vi "read data.vi"(0 "Control ref":refnum<vi>, 2 "Data In":T1, 4 "index":i32, 5 "error in (no error)":errorcluster) -> ()   [LabVIEW 2014, in "X DIM conditions.xctl"]
uses:
  X DIM conditions.xctl
  X DIM conditions.Data.ctl
  PTSequencer/PTSequencer.DIM service condition.ctl
  CSCore/CSSystem/CoreDefs/CoreDefs.rawDataType.ctl
  CSCore/CSSystem/CoreLib/CoreLib.byte array 2 string.vi
  CSCore/CSSystem/CoreLib/CoreLib.byte array 2 int.vi
  CSCore/CSSystem/CoreLib/CoreLib.byte array 2 int array.vi
  CSCore/CSSystem/CoreLib/CoreLib.byte array 2 short.vi
  CSCore/CSSystem/CoreLib/CoreLib.byte array 2 short array.vi
  CSCore/CSSystem/CoreLib/CoreLib.byte array 2 double.vi
  CSCore/CSSystem/CoreLib/CoreLib.byte array 2 double array.vi
  CSCore/CSSystem/CoreLib/CoreLib.byte array 2 float.vi
  CSCore/CSSystem/CoreLib/CoreLib.byte array 2 float array.vi
  CSCore/CSSystem/CoreLib/CoreLib.lvlib
  PTSequencer/PTSequencer.lvlib
panel:
  in  "Control":T4
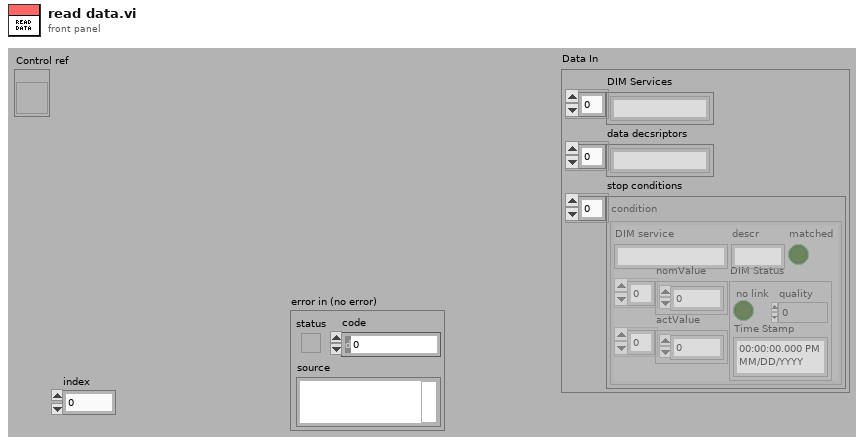
[diagram p1: front panel]
types:
  T1 = typedef "X DIM conditions.xctl/X DIM conditions.Data.ctl" = cluster{"DIM Services":string[], "data decsriptors":string[], "stop conditions":T2[]}
  T2 = typedef "PTSequencer.lvlib/PTSequencer.DIM service condition.ctl" = cluster{"DIM service":string, "descr":string, "nomValue":T3, "actValue":T3, "matched":bool, "DIM Status":cluster{"no link":bool, "quality":i32, "Time Stamp":timestamp}}
  T3 = typedef "CoreDefs.rawDataType.ctl" = i8[]
  T4 = cluster{"Name 1":u16, "Descr 1":string, "Value 1":string, "Used 1":bool, "Name 2":u16, "Descr 2":string, "Value 2":string, "Used 2":bool, "Name 3":u16, "Descr 3":string, "Value 3":string, "Used 3":bool, "Name 4":u16, "Descr 4":string, "Value 4":string, "Used 4":bool}
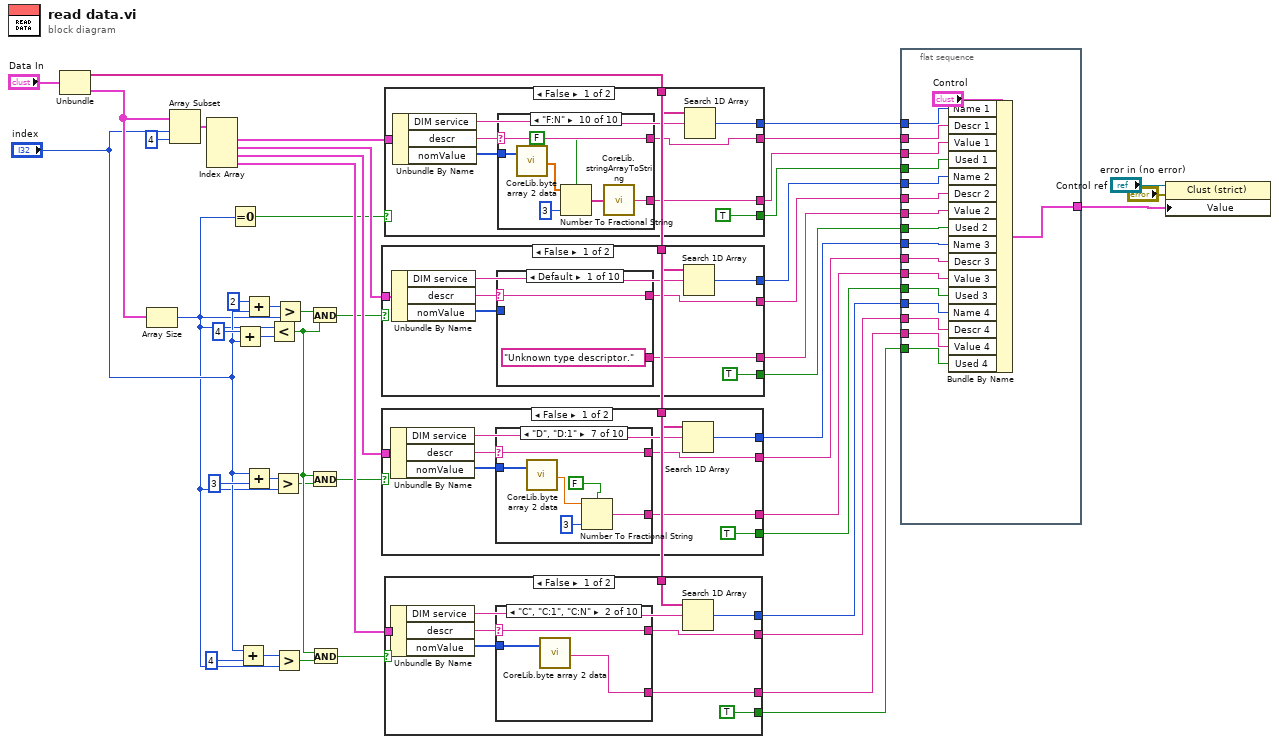
[diagram p0: block diagram]
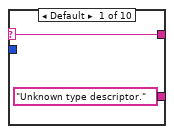
[diagram p2: hidden frame]
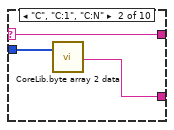
[diagram p3: hidden frame]
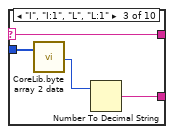
[diagram p4: hidden frame]
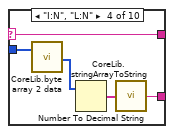
[diagram p5: hidden frame]
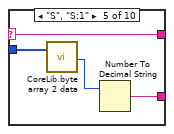
[diagram p6: hidden frame]
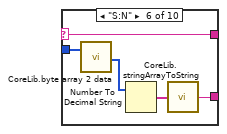
[diagram p7: hidden frame]
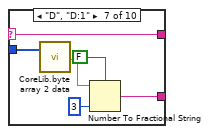
[diagram p8: hidden frame]
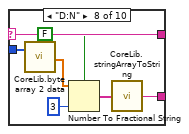
[diagram p9: hidden frame]
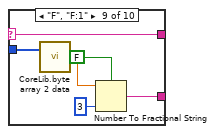
[diagram p10: hidden frame]
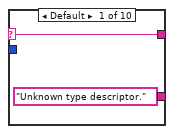
[diagram p12: hidden frame]
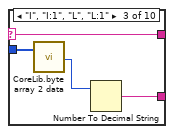
[diagram p13: hidden frame]
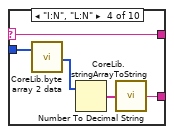
[diagram p14: hidden frame]
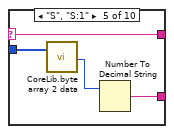
[diagram p15: hidden frame]
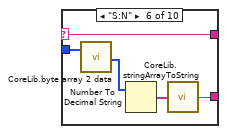
[diagram p16: hidden frame]
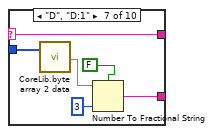
[diagram p17: hidden frame]
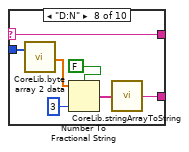
[diagram p18: hidden frame]
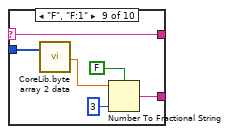
[diagram p19: hidden frame]
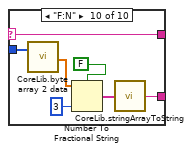
[diagram p20: hidden frame]
diagram:
  n1 = Unbundle("Data In") -> ("DIM Services"=w24:string[], "stop conditions"=w23:T2[])  [unwired: 1 out]
  n2 = Array Size(array=w23) -> (size(s)=w2:i32)
  n3 = Array Subset(array=w23, index="index", length=4) -> (w45:T2[])
  n4 = Index Array(array=w45) -> (element #1=w44:T2, element #2=w43:T2, element #3=w42:T2, element #4=w41:T2)  [unwired: 4 in]
  n5 = Equal To 0?(x=w2) -> (x = 0?=w1:bool)
  n6 = Add(x=4, y="index") -> (x+y=w15:i32)
  n7 = Add(x="index", y=4) -> (x+y=w19:i32)
  n8 = Add(x=2, y="index") -> (x+y=w16:i32)
  n9 = Add(x="index", y=3) -> (x+y=w18:i32)
  n10 = Less?(x=w2, y=w15) -> (x < y?=w13:bool)
  n11 = Greater?(x=w18, y=w2) -> (0:w11:bool)
  n12 = Greater?(x=w19, y=w2) -> (0:w12:bool)
  n13 = Greater?(x=w16, y=w2) -> (0:w10:bool)
  n14 = And(x=w10, y=w13) -> (x .and. y?=w6:bool)
  n15 = And(x=w13, y=w11) -> (x .and. y?=w7:bool)
  n16 = And(x=w13, y=w12) -> (x .and. y?=w8:bool)
  n17 = case shown="False" w6 {
    tunnel: w43 -> [w52 _]
    tunnel: [w51 _] -> w39
    tunnel: [w50 _] -> w37
    tunnel: [w49 _] -> w36
    tunnel: w24 -> [w48 _]
    tunnel: [TRUE _] -> w5
    frame False {
      n18 = Unbundle By Name(w52) -> ("DIM service"=w55:string, "descr"=w53:string, "nomValue"=w54:T3)
      n19 = case shown="Default" w53 {
        selector: w53 -> [w56 w58 w61 w65 w70 w74 w83 w87 w96 w100]
        tunnel: w54 -> [_ w60 w64 w69 w73 w78 w84 w91 w97 w102]
        tunnel: ["Unknown type descriptor." w59 w62 w66 w71 w75 w81 w88 w94 w101] -> w49
        tunnel: [w56 w58 w61 w65 w70 w74 w83 w87 w96 w100] -> w50
        frame Default {
        }
        frame "C", "C:1", "C:N" {
          n20 = call-poly "CoreLib.byte array 2 data.vi"("byteArray"=w60) -> ("string"=w59:string)  [unwired: 16 in, 2 out]
        }
        frame "I", "I:1", "L", "L:1" {
          n21 = call-poly "CoreLib.byte array 2 data.vi"("byteArray"=w64) -> ("i32"=w63:i32)  [unwired: 16 in, 2 out]
          n22 = Number To Decimal String(number=w63) -> (decimal integer string=w62:string)  [unwired: 1 in]
        }
        frame "I:N", "L:N" {
          n23 = call-poly "CoreLib.byte array 2 data.vi"("byteArray"=w69) -> ("[i32]"=w68:i32[])  [unwired: 16 in, 2 out]
          n24 = Number To Decimal String(number=w68) -> (decimal integer string=w67:string[])  [unwired: 1 in]
          n25 = call "CoreLib.stringArrayToString.vi"("Array"=w67) -> ("String"=w66:string)
        }
        frame "S", "S:1" {
          n26 = call-poly "CoreLib.byte array 2 data.vi"("byteArray"=w73) -> ("i16"=w72:i16)  [unwired: 16 in, 2 out]
          n27 = Number To Decimal String(number=w72) -> (decimal integer string=w71:string)  [unwired: 1 in]
        }
        frame "S:N" {
          n28 = call-poly "CoreLib.byte array 2 data.vi"("byteArray"=w78) -> ("[i16]"=w77:i16[])  [unwired: 16 in, 2 out]
          n29 = Number To Decimal String(number=w77) -> (decimal integer string=w76:string[])  [unwired: 1 in]
          n30 = call "CoreLib.stringArrayToString.vi"("Array"=w76) -> ("String"=w75:string)
        }
        frame "D", "D:1" {
          n31 = call-poly "CoreLib.byte array 2 data.vi"("byteArray"=w84) -> ("d64"=w80:dbl)  [unwired: 16 in, 2 out]
          n32 = Number To Fractional String(use system decimal point (T)=FALSE, number=w80, precision (6)=i16 3) -> (F-format string=w81:string)  [unwired: 1 in]
        }
        frame "D:N" {
          n33 = call-poly "CoreLib.byte array 2 data.vi"("byteArray"=w91) -> ("[d64]"=w90:dbl[])  [unwired: 16 in, 2 out]
          n34 = Number To Fractional String(use system decimal point (T)=FALSE, number=w90, precision (6)=i16 3) -> (F-format string=w89:string[])  [unwired: 1 in]
          n35 = call "CoreLib.stringArrayToString.vi"("Array"=w89) -> ("String"=w88:string)
        }
        frame "F", "F:1" {
          n36 = call-poly "CoreLib.byte array 2 data.vi"("byteArray"=w97) -> ("f32"=w93:sgl)  [unwired: 16 in, 2 out]
          n37 = Number To Fractional String(use system decimal point (T)=FALSE, number=w93, precision (6)=i16 3) -> (F-format string=w94:string)  [unwired: 1 in]
        }
        frame "F:N" {
          n38 = call-poly "CoreLib.byte array 2 data.vi"("byteArray"=w102) -> ("[f32]"=w104:sgl[])  [unwired: 16 in, 2 out]
          n39 = Number To Fractional String(use system decimal point (T)=FALSE, number=w104, precision (6)=i16 3) -> (F-format string=w103:string[])  [unwired: 1 in]
          n40 = call "CoreLib.stringArrayToString.vi"("Array"=w103) -> ("String"=w101:string)
        }
      }
      n41 = Search 1D Array(1D array=w48, element=w55) -> (index of element=w51:i32)  [unwired: 1 in]
    }
    frame True {
    }
  }
  n42 = case shown="False" w7 {
    tunnel: w42 -> [w110 _]
    tunnel: [w109 _] -> w38
    tunnel: [w108 _] -> w35
    tunnel: [w107 _] -> w34
    tunnel: w24 -> [w106 _]
    tunnel: [TRUE _] -> w4
    frame False {
      n43 = Unbundle By Name(w110) -> ("DIM service"=w111:string, "descr"=w113:string, "nomValue"=w112:T3)
      n44 = case shown="\"D\", \"D:1\"" w113 {
        selector: w113 -> [w114 w116 w119 w123 w128 w132 w141 w145 w154 w158]
        tunnel: w112 -> [_ w118 w122 w127 w131 w136 w142 w149 w155 w160]
        tunnel: ["Unknown type descriptor." w117 w120 w124 w129 w133 w138 w146 w152 w159] -> w107
        tunnel: [w114 w116 w119 w123 w128 w132 w141 w145 w154 w158] -> w108
        frame Default {
        }
        frame "C", "C:1", "C:N" {
          n45 = call-poly "CoreLib.byte array 2 data.vi"("byteArray"=w118) -> ("string"=w117:string)  [unwired: 16 in, 2 out]
        }
        frame "I", "I:1", "L", "L:1" {
          n46 = call-poly "CoreLib.byte array 2 data.vi"("byteArray"=w122) -> ("i32"=w121:i32)  [unwired: 16 in, 2 out]
          n47 = Number To Decimal String(number=w121) -> (decimal integer string=w120:string)  [unwired: 1 in]
        }
        frame "I:N", "L:N" {
          n48 = call-poly "CoreLib.byte array 2 data.vi"("byteArray"=w127) -> ("[i32]"=w126:i32[])  [unwired: 16 in, 2 out]
          n49 = Number To Decimal String(number=w126) -> (decimal integer string=w125:string[])  [unwired: 1 in]
          n50 = call "CoreLib.stringArrayToString.vi"("Array"=w125) -> ("String"=w124:string)
        }
        frame "S", "S:1" {
          n51 = call-poly "CoreLib.byte array 2 data.vi"("byteArray"=w131) -> ("i16"=w130:i16)  [unwired: 16 in, 2 out]
          n52 = Number To Decimal String(number=w130) -> (decimal integer string=w129:string)  [unwired: 1 in]
        }
        frame "S:N" {
          n53 = call-poly "CoreLib.byte array 2 data.vi"("byteArray"=w136) -> ("[i16]"=w135:i16[])  [unwired: 16 in, 2 out]
          n54 = Number To Decimal String(number=w135) -> (decimal integer string=w134:string[])  [unwired: 1 in]
          n55 = call "CoreLib.stringArrayToString.vi"("Array"=w134) -> ("String"=w133:string)
        }
        frame "D", "D:1" {
          n56 = call-poly "CoreLib.byte array 2 data.vi"("byteArray"=w142) -> ("d64"=w139:dbl)  [unwired: 16 in, 2 out]
          n57 = Number To Fractional String(use system decimal point (T)=FALSE, number=w139, precision (6)=i16 3) -> (F-format string=w138:string)  [unwired: 1 in]
        }
        frame "D:N" {
          n58 = call-poly "CoreLib.byte array 2 data.vi"("byteArray"=w149) -> ("[d64]"=w148:dbl[])  [unwired: 16 in, 2 out]
          n59 = Number To Fractional String(use system decimal point (T)=FALSE, number=w148, precision (6)=i16 3) -> (F-format string=w147:string[])  [unwired: 1 in]
          n60 = call "CoreLib.stringArrayToString.vi"("Array"=w147) -> ("String"=w146:string)
        }
        frame "F", "F:1" {
          n61 = call-poly "CoreLib.byte array 2 data.vi"("byteArray"=w155) -> ("f32"=w151:sgl)  [unwired: 16 in, 2 out]
          n62 = Number To Fractional String(use system decimal point (T)=FALSE, number=w151, precision (6)=i16 3) -> (F-format string=w152:string)  [unwired: 1 in]
        }
        frame "F:N" {
          n63 = call-poly "CoreLib.byte array 2 data.vi"("byteArray"=w160) -> ("[f32]"=w162:sgl[])  [unwired: 16 in, 2 out]
          n64 = Number To Fractional String(use system decimal point (T)=FALSE, number=w162, precision (6)=i16 3) -> (F-format string=w161:string[])  [unwired: 1 in]
          n65 = call "CoreLib.stringArrayToString.vi"("Array"=w161) -> ("String"=w159:string)
        }
      }
      n66 = Search 1D Array(1D array=w106, element=w111) -> (index of element=w109:i32)  [unwired: 1 in]
    }
    frame True {
    }
  }
  n67 = case shown="False" w1 {
    tunnel: w44 -> [w168 _]
    tunnel: [w167 _] -> w40
    tunnel: [w166 _] -> w33
    tunnel: [w165 _] -> w32
    tunnel: w24 -> [w164 _]
    tunnel: [TRUE _] -> w22
    frame False {
      n68 = Unbundle By Name(w168) -> ("DIM service"=w169:string, "descr"=w171:string, "nomValue"=w170:T3)
      n69 = case shown="\"F:N\"" w171 {
        selector: w171 -> [w172 w174 w177 w181 w186 w190 w199 w203 w212 w216]
        tunnel: w170 -> [_ w176 w180 w185 w189 w194 w200 w207 w213 w218]
        tunnel: ["Unknown type descriptor." w175 w178 w182 w187 w191 w198 w204 w210 w217] -> w166
        tunnel: [w172 w174 w177 w181 w186 w190 w199 w203 w212 w216] -> w165
        frame Default {
        }
        frame "C", "C:1", "C:N" {
          n70 = call-poly "CoreLib.byte array 2 data.vi"("byteArray"=w176) -> ("string"=w175:string)  [unwired: 16 in, 2 out]
        }
        frame "I", "I:1", "L", "L:1" {
          n71 = call-poly "CoreLib.byte array 2 data.vi"("byteArray"=w180) -> ("i32"=w179:i32)  [unwired: 16 in, 2 out]
          n72 = Number To Decimal String(number=w179) -> (decimal integer string=w178:string)  [unwired: 1 in]
        }
        frame "I:N", "L:N" {
          n73 = call-poly "CoreLib.byte array 2 data.vi"("byteArray"=w185) -> ("[i32]"=w184:i32[])  [unwired: 16 in, 2 out]
          n74 = Number To Decimal String(number=w184) -> (decimal integer string=w183:string[])  [unwired: 1 in]
          n75 = call "CoreLib.stringArrayToString.vi"("Array"=w183) -> ("String"=w182:string)
        }
        frame "S", "S:1" {
          n76 = call-poly "CoreLib.byte array 2 data.vi"("byteArray"=w189) -> ("i16"=w188:i16)  [unwired: 16 in, 2 out]
          n77 = Number To Decimal String(number=w188) -> (decimal integer string=w187:string)  [unwired: 1 in]
        }
        frame "S:N" {
          n78 = call-poly "CoreLib.byte array 2 data.vi"("byteArray"=w194) -> ("[i16]"=w193:i16[])  [unwired: 16 in, 2 out]
          n79 = Number To Decimal String(number=w193) -> (decimal integer string=w192:string[])  [unwired: 1 in]
          n80 = call "CoreLib.stringArrayToString.vi"("Array"=w192) -> ("String"=w191:string)
        }
        frame "D", "D:1" {
          n81 = call-poly "CoreLib.byte array 2 data.vi"("byteArray"=w200) -> ("d64"=w196:dbl)  [unwired: 16 in, 2 out]
          n82 = Number To Fractional String(use system decimal point (T)=FALSE, number=w196, precision (6)=i16 3) -> (F-format string=w198:string)  [unwired: 1 in]
        }
        frame "D:N" {
          n83 = call-poly "CoreLib.byte array 2 data.vi"("byteArray"=w207) -> ("[d64]"=w206:dbl[])  [unwired: 16 in, 2 out]
          n84 = Number To Fractional String(use system decimal point (T)=FALSE, number=w206, precision (6)=i16 3) -> (F-format string=w205:string[])  [unwired: 1 in]
          n85 = call "CoreLib.stringArrayToString.vi"("Array"=w205) -> ("String"=w204:string)
        }
        frame "F", "F:1" {
          n86 = call-poly "CoreLib.byte array 2 data.vi"("byteArray"=w213) -> ("f32"=w211:sgl)  [unwired: 16 in, 2 out]
          n87 = Number To Fractional String(use system decimal point (T)=FALSE, number=w211, precision (6)=i16 3) -> (F-format string=w210:string)  [unwired: 1 in]
        }
        frame "F:N" {
          n88 = call-poly "CoreLib.byte array 2 data.vi"("byteArray"=w218) -> ("[f32]"=w220:sgl[])  [unwired: 16 in, 2 out]
          n89 = Number To Fractional String(use system decimal point (T)=FALSE, number=w220, precision (6)=i16 3) -> (F-format string=w219:string[])  [unwired: 1 in]
          n90 = call "CoreLib.stringArrayToString.vi"("Array"=w219) -> ("String"=w217:string)
        }
      }
      n91 = Search 1D Array(1D array=w164, element=w169) -> (index of element=w167:i32)  [unwired: 1 in]
    }
    frame True {
    }
  }
  n92 = case shown="False" w8 {
    tunnel: w41 -> [w226 _]
    tunnel: [w225 _] -> w31
    tunnel: [w224 _] -> w30
    tunnel: [w223 _] -> w29
    tunnel: w24 -> [w222 _]
    tunnel: [TRUE _] -> w3
    frame False {
      n93 = Unbundle By Name(w226) -> ("DIM service"=w229:string, "descr"=w227:string, "nomValue"=w228:T3)
      n94 = case shown="\"C\", \"C:1\", \"C:N\"" w227 {
        selector: w227 -> [w230 w232 w235 w239 w244 w248 w257 w261 w270 w274]
        tunnel: w228 -> [_ w234 w238 w243 w247 w252 w258 w265 w271 w276]
        tunnel: ["Unknown type descriptor." w233 w236 w240 w245 w249 w255 w262 w268 w275] -> w223
        tunnel: [w230 w232 w235 w239 w244 w248 w257 w261 w270 w274] -> w224
        frame Default {
        }
        frame "C", "C:1", "C:N" {
          n95 = call-poly "CoreLib.byte array 2 data.vi"("byteArray"=w234) -> ("string"=w233:string)  [unwired: 16 in, 2 out]
        }
        frame "I", "I:1", "L", "L:1" {
          n96 = call-poly "CoreLib.byte array 2 data.vi"("byteArray"=w238) -> ("i32"=w237:i32)  [unwired: 16 in, 2 out]
          n97 = Number To Decimal String(number=w237) -> (decimal integer string=w236:string)  [unwired: 1 in]
        }
        frame "I:N", "L:N" {
          n98 = call-poly "CoreLib.byte array 2 data.vi"("byteArray"=w243) -> ("[i32]"=w242:i32[])  [unwired: 16 in, 2 out]
          n99 = Number To Decimal String(number=w242) -> (decimal integer string=w241:string[])  [unwired: 1 in]
          n100 = call "CoreLib.stringArrayToString.vi"("Array"=w241) -> ("String"=w240:string)
        }
        frame "S", "S:1" {
          n101 = call-poly "CoreLib.byte array 2 data.vi"("byteArray"=w247) -> ("i16"=w246:i16)  [unwired: 16 in, 2 out]
          n102 = Number To Decimal String(number=w246) -> (decimal integer string=w245:string)  [unwired: 1 in]
        }
        frame "S:N" {
          n103 = call-poly "CoreLib.byte array 2 data.vi"("byteArray"=w252) -> ("[i16]"=w251:i16[])  [unwired: 16 in, 2 out]
          n104 = Number To Decimal String(number=w251) -> (decimal integer string=w250:string[])  [unwired: 1 in]
          n105 = call "CoreLib.stringArrayToString.vi"("Array"=w250) -> ("String"=w249:string)
        }
        frame "D", "D:1" {
          n106 = call-poly "CoreLib.byte array 2 data.vi"("byteArray"=w258) -> ("d64"=w254:dbl)  [unwired: 16 in, 2 out]
          n107 = Number To Fractional String(use system decimal point (T)=FALSE, number=w254, precision (6)=i16 3) -> (F-format string=w255:string)  [unwired: 1 in]
        }
        frame "D:N" {
          n108 = call-poly "CoreLib.byte array 2 data.vi"("byteArray"=w265) -> ("[d64]"=w264:dbl[])  [unwired: 16 in, 2 out]
          n109 = Number To Fractional String(use system decimal point (T)=FALSE, number=w264, precision (6)=i16 3) -> (F-format string=w263:string[])  [unwired: 1 in]
          n110 = call "CoreLib.stringArrayToString.vi"("Array"=w263) -> ("String"=w262:string)
        }
        frame "F", "F:1" {
          n111 = call-poly "CoreLib.byte array 2 data.vi"("byteArray"=w271) -> ("f32"=w267:sgl)  [unwired: 16 in, 2 out]
          n112 = Number To Fractional String(use system decimal point (T)=FALSE, number=w267, precision (6)=i16 3) -> (F-format string=w268:string)  [unwired: 1 in]
        }
        frame "F:N" {
          n113 = call-poly "CoreLib.byte array 2 data.vi"("byteArray"=w276) -> ("[f32]"=w278:sgl[])  [unwired: 16 in, 2 out]
          n114 = Number To Fractional String(use system decimal point (T)=FALSE, number=w278, precision (6)=i16 3) -> (F-format string=w277:string[])  [unwired: 1 in]
          n115 = call "CoreLib.stringArrayToString.vi"("Array"=w277) -> ("String"=w275:string)
        }
      }
      n116 = Search 1D Array(1D array=w222, element=w229) -> (index of element=w225:i32)  [unwired: 1 in]
    }
    frame True {
    }
  }
  n117 = flat-sequence {
    tunnel: w40 -> [w284]
    tunnel: w39 -> [w287]
    tunnel: w38 -> [w286]
    tunnel: w37 -> [w296]
    tunnel: w36 -> [w295]
    tunnel: w35 -> [w294]
    tunnel: w34 -> [w293]
    tunnel: w33 -> [w292]
    tunnel: w32 -> [w291]
    tunnel: w31 -> [w285]
    tunnel: w30 -> [w290]
    tunnel: w29 -> [w289]
    tunnel: [w288] -> w28
    tunnel: w22 -> [w282]
    tunnel: w5 -> [w281]
    tunnel: w4 -> [w280]
    tunnel: w3 -> [w279]
    frame #0 {
      n118 = Bundle By Name(cluster="Control", "Name 1"=w284, "Descr 1"=w291, "Value 1"=w292, "Used 1"=w282, "Name 2"=w287, "Descr 2"=w296, "Value 2"=w295, "Used 2"=w281, "Name 3"=w286, "Descr 3"=w294, "Value 3"=w293, "Used 3"=w280, "Name 4"=w285, "Descr 4"=w290, "Value 4"=w289, "Used 4"=w279) -> (w288:T4)
    }
  }
  n119 = property class="Clust (strict)"(reference="Control ref", error in="error in (no error)", "Value"=w28) -> ()  [unwired: 2 out]
